vi "2898 Dashboard Send.vi"   [LabVIEW 2011]
uses:
  Team Code/Robot Global Data.vi
types:
  T1 = typedef "Dashboard Data TypeDef.ctl" = cluster{"Number of Balls":i32, "Shooting Manual Override?":bool, "Bridge Mode?":bool, "Shooter":bool, "Shooter At Speed?":bool, "Aligning Mode?":bool}
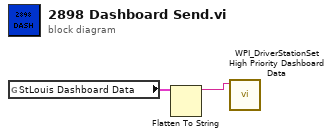
[diagram p0: block diagram]
diagram:
  n1 = global read "Robot Global Data.vi" "StLouis Dashboard Data"() -> (w2:T1)
  n2 = Flatten To String(anything=w2) -> (data string=w1:string)  [unwired: 3 in, 2 out]
  n3 = call <vilib>:"WPI_DriverStationSet High Priority Dashboard Data.vi"("User Data"=w1) -> ()  [unwired: 10 in, 1 out]
